vi "subUpdateCSharpProjectFile.vi"(8 "error in (no error)":errorcluster, 11 ".csproj path":path) -> (0 "error out":errorcluster, 3 ".csproj path out":path)   [LabVIEW 2015, in "veristand-steps-codegen.lvlib"]
uses:
  veristand-steps-codegen.lvlib
  <vilib>/xml/Load XML File.vi
  <vilib>/xml/Close Reference(Node).vi
  <vilib>/xml/Close Reference(NNMap).vi
  <vilib>/ni/Simple XML/_polymorphics/Create Tag - Child with Text.vi
  <vilib>/xml/NI_XML.lvlib
  <resource>/objmgr/DOMUserDefRef.rc
  <vilib>/ni/Simple XML/Simple XML.lvlib
panel:
  out "error out":errorcluster
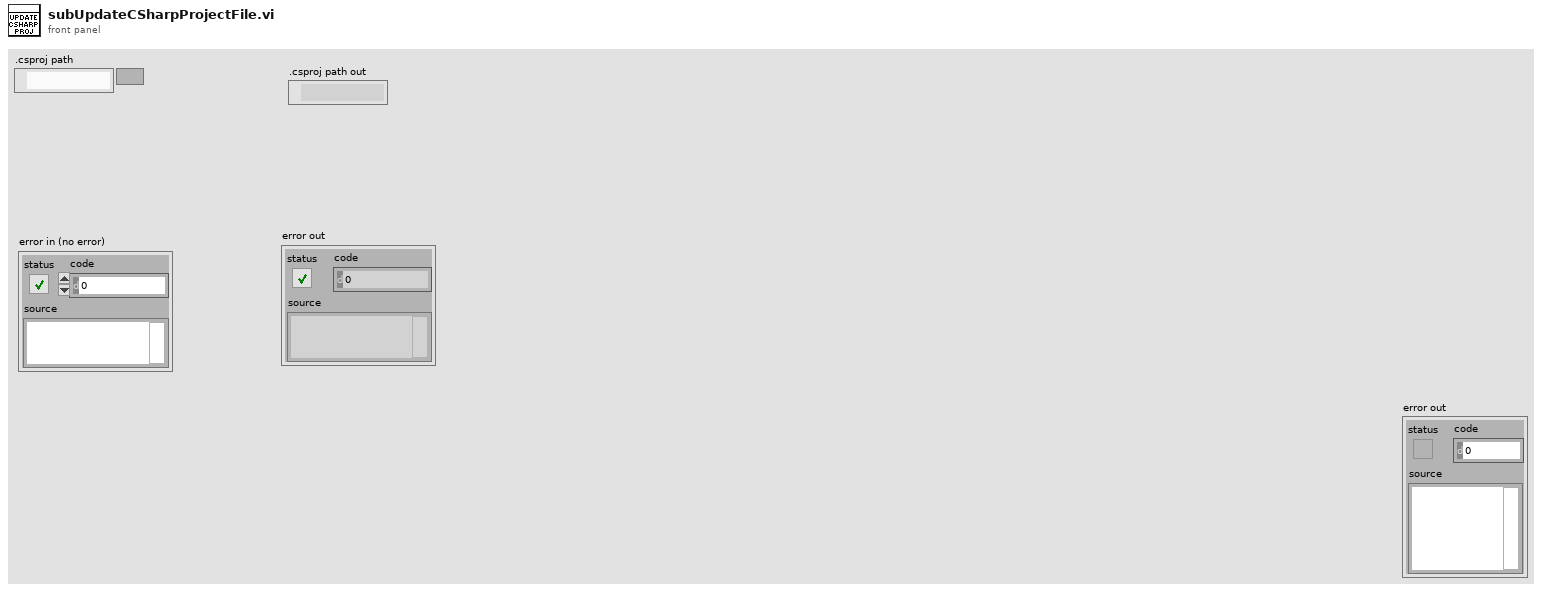
[diagram p1: front panel]
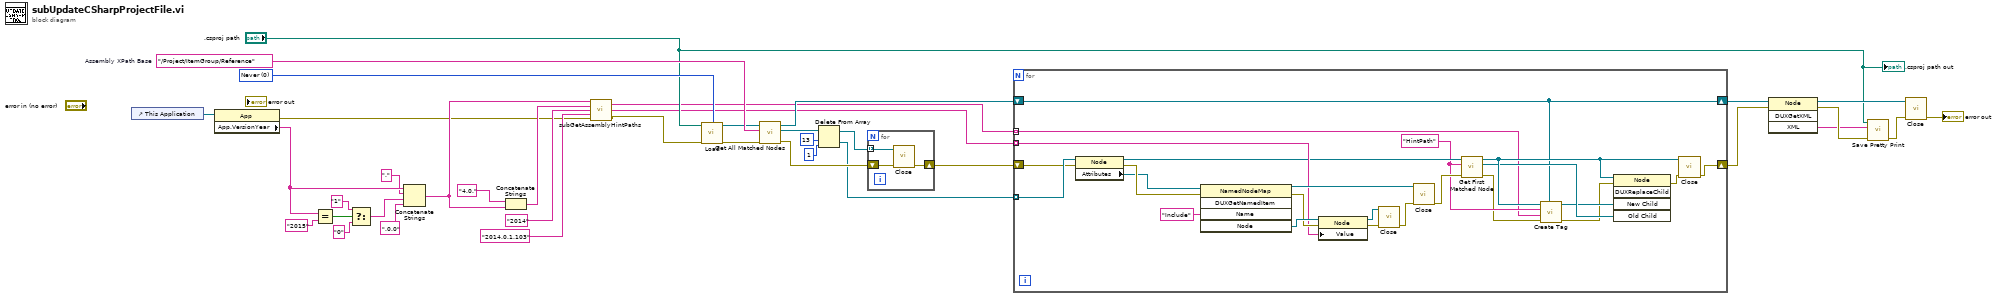
[diagram p0: block diagram]
diagram:
  w23 = "/Project/ItemGroup/Reference"  # Assembly XPath Base
  w20 = 0 items=["Never", "Always", "Auto"] ("validate on load (Auto)")
  n1 = control-ref of="This Application"() -> (w15:refnum<vi>)
  n2 = property class="App"(reference=w15) -> (error out=w1:errorcluster, "App.VersionYear"=w12:string)  [unwired: 1 in, 1 out]
  n3 = Equal?(x=w12, y="2015") -> (x = y?=w10:bool)
  n4 = Select(t="1" ("string"), s=w10, f="0" ("string")) -> (s? t:f=w7:string)
  n5 = Concatenate Strings(w12, "." ("string"), w7, ".0.0" ("string")) -> (w4:string)
  n6 = Concatenate Strings("4.0." ("string"), w4) -> (w2:string)
  n7 = call "subGetAssemblyHintPaths.vi"("VeriStand assembly version string (2014.0.0.0)"=w4, "VeriStand GAC assembly version (4.0.2014.0.0.0)"=w2, "TestStand version string (2014)"="2014", "TestStand assembly version (2014.0.0.0)"="2014.0.1.103", "error in"=w1) -> ("New Assembly Hint Paths"=w16:string[], "New Assembly Include Paths"=w17:string[], "error out"=w18:errorcluster)  [unwired: 8 in]
  n8 = call-poly <vilib>:"Load.vi"("path to XML document"=".csproj path", "validate on load (Auto)"=w20, "error in (no error)"=w18) -> ("DOM document out"=w22:refnum<k20>, "error out"=w21:errorcluster)  [unwired: 10 in, 1 out]
  n9 = call <vilib>:"Get All Matched Nodes.vi"("error in (no error)"=w21, "XPath expression"=w23, "node in"=w22) -> ("error out"=w29:errorcluster, "node result array"=w24:refnum<k20>[], "node out"=w36:refnum<k20>)  [unwired: 6 in]
  n10 = Delete From Array(array=w24, length=13, index=1 ("length")) -> (deleted portion=w27:refnum<k20>[], array with subset deleted=w28:refnum<k20>[])
  n11 = for {
    tunnel: w28 -> [w41] mode=indexing
    shift-right: [w39] -> w30
    shift-left: w29 -> [w40]
    n12 = call-poly <vilib>:"Close.vi"("error in (no error)"=w40, "node"=w41) -> ("error out"=w39:errorcluster)  [unwired: 7 in]
  }
  n13 = for {
    tunnel: w27 -> [w62] mode=indexing
    shift-right: [w56] -> w31
    shift-left: w30 -> [w61]
    tunnel: w17 -> [w55] mode=indexing
    tunnel: w16 -> [w43] mode=indexing
    shift-right: [w42] -> w37
    shift-left: w36 -> [w42]
    w50 = "HintPath" ("XPath expression")
    n14 = property class="Node"(reference=w62, error in=w61) -> (reference out=w51:refnum<k20>, error out=w65:errorcluster, "Attributes"=w63:refnum<k20>)
    n15 = invoke class="NamedNodeMap" method="DUXGetNamedItem"(reference=w63, error in=w65, "Name"="Include") -> (reference out=w57:refnum<k20>, error out=w59:errorcluster, "Node"=w60:refnum<k20>)  [unwired: 2 in, 2 out]
    n16 = property class="Node"(reference=w60, error in=w59, "Value"=w55) -> (reference out=w58:refnum<k20>, error out=w54:errorcluster)
    n17 = call-poly <vilib>:"Close.vi"("error in (no error)"=w54, "node"=w58) -> ("error out"=w53:errorcluster)  [unwired: 7 in]
    n18 = call-poly <vilib>:"Close.vi"("error in (no error)"=w53, "named node map"=w57) -> ("error out"=w52:errorcluster)  [unwired: 7 in]
    n19 = call <vilib>:"Get First Matched Node.vi"("error in (no error)"=w52, "XPath expression"=w50, "node in"=w51) -> ("error out"=w49:errorcluster, "node result"=w47:refnum<k20>, "node out"=w48:refnum<k20>)  [unwired: 6 in]
    n20 = call-poly <vilib>:"Create Tag.vi"("DOM document reference"=w42, "error in (no error)"=w49, "Text Data"=w43, "Tag Name"=w50, "Parent Element reference"=w48) -> ("error out"=w45:errorcluster, "Child Element reference"=w46:refnum<k20>)  [unwired: 5 in]
    n21 = invoke class="Node" method="DUXReplaceChild"(reference=w48, error in=w45, "New Child"=w46, "Old Child"=w47) -> (error out=w44:errorcluster)  [unwired: 1 in, 4 out]
    n22 = call-poly <vilib>:"Close.vi"("error in (no error)"=w44, "node"=w48) -> ("error out"=w56:errorcluster)  [unwired: 7 in]
  }
  n23 = invoke class="Node" method="DUXGetXML"(reference=w37, error in=w31) -> (reference out=w35:refnum<k20>, error out=w33:errorcluster, "XML"=w32:string)  [unwired: 2 in, 1 out]
  n24 = call <vilib>:"Save Pretty Print.vi"("error in (no error)"=w33, "Pretty XML String"=w32, "XML file path"=".csproj path") -> ("error out"=w34:errorcluster)  [unwired: 7 in, 1 out]
  n25 = call-poly <vilib>:"Close.vi"("error in (no error)"=w34, "node"=w35) -> ("error out"=→"error out":errorcluster)  [unwired: 7 in]
  ".csproj path out" <- ".csproj path"
